vi "VF Laser Engine.vi"(0 "VF Laser Notifier":string="Not a Name", 11 "COM Port":string[](array[string])) -> ()   [LabVIEW 2020]
uses:
  Laser Controls/Laser Status.ctl
  Laser Controls/Laser Notifier Element.ctl
  Laser Controls/Laser Actions.ctl
  Laser Controls/Laser Settings.ctl
  Laser Controls/Laser Parameters.ctl
  <vilib>/Instr/_visa.llb/VISA Configure Serial Port (Instr).vi
panel:
  out "Startup Error":errorcluster
  in  "Get Power":bool
  out "Status":T1
  out "Light Emission?":bool
  out "Enabled (Interlock)?":bool
  in  "Get Status":bool
  in  "Laser Power (mW)":dbl
  in  "Laser On/Off":bool
  in  "Quit":bool
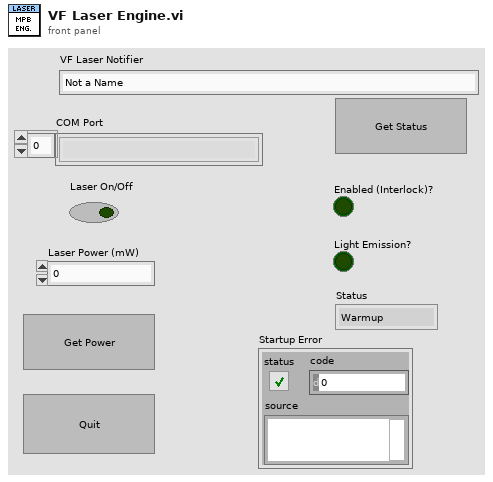
[diagram p1: front panel]
types:
  T1 = typedef "Laser Status.ctl" = enum16{"Warmup", "Ready", "Emission", "Tuning", "Error"}
  T2 = typedef "Laser Notifier Element.ctl" = cluster{"Laser Action":T3, "Received?":bool, "Enabled (Interlock)?":bool, "Light Emission?":bool, "Power (mW)":dbl, "Settings":T4, "Status":T1, "Error":errorcluster}
  T3 = typedef "Laser Actions.ctl" = enum16{"Error Check", "Set On/Off", "Set Power", "Set Parameter", "Get Power", "Get Status", "Get Parameter", "Quit"}
  T4 = typedef "Laser Settings.ctl" = cluster{"Laser Parameters":T5, "Value":dbl}
  T5 = typedef "Laser Parameters.ctl" = enum16{"Wavelength (nm)", "Pulsing?", "Rep. Rate", "External Control"}
  T6 = enum32{"Invalid", "Standard", "Closed", "Hidden", "Minimized", "Maximized"}
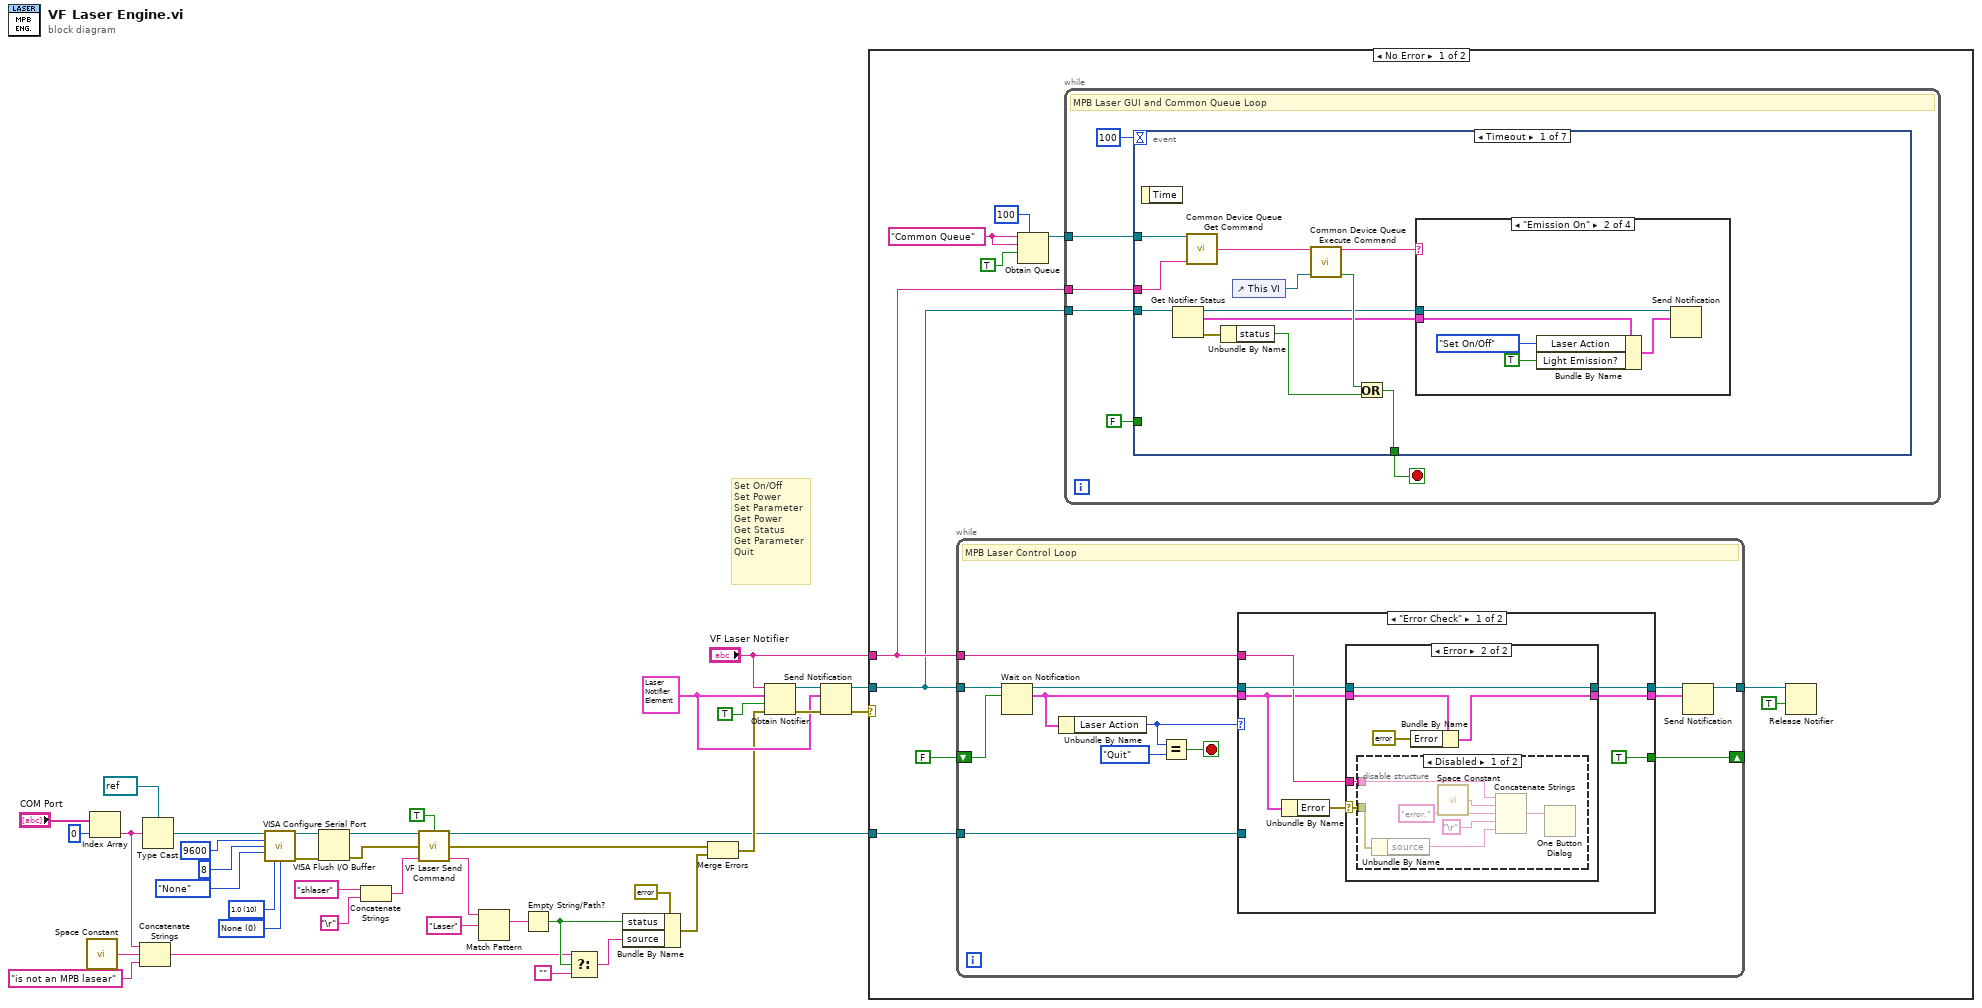
[diagram p0: block diagram]
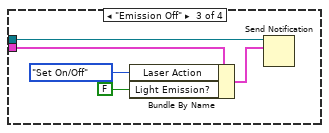
[diagram p3: hidden frame]
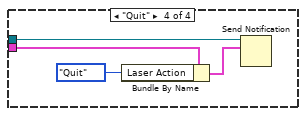
[diagram p4: hidden frame]
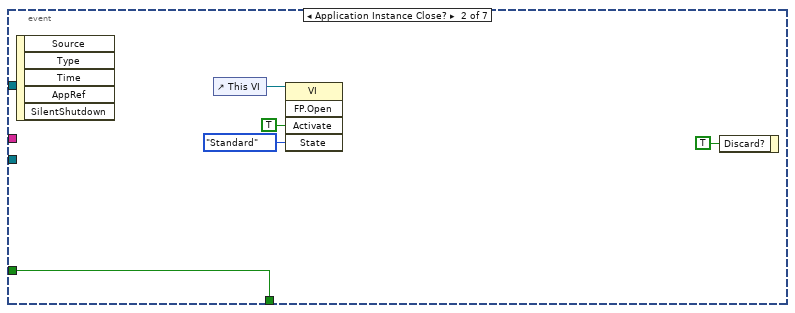
[diagram p5: hidden frame]
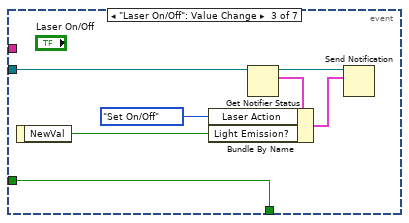
[diagram p6: hidden frame]
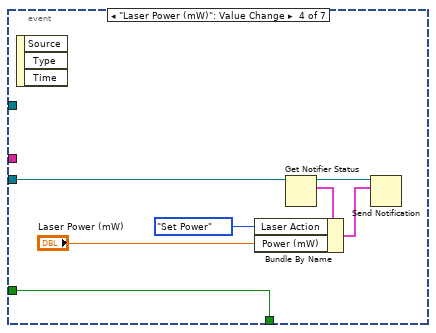
[diagram p7: hidden frame]
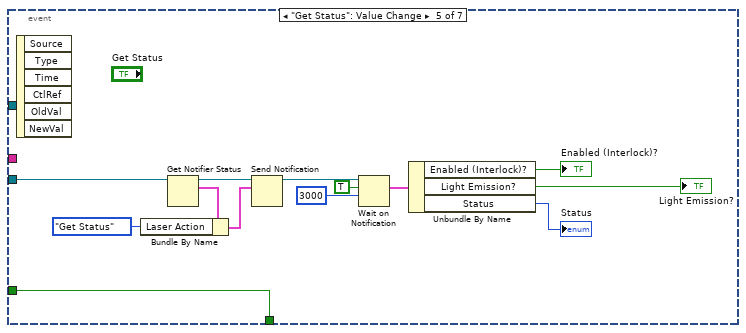
[diagram p8: hidden frame]
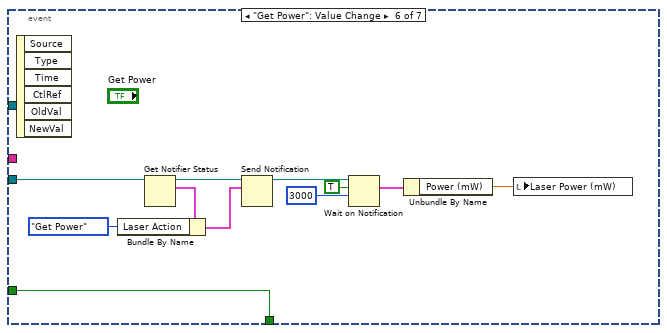
[diagram p9: hidden frame]
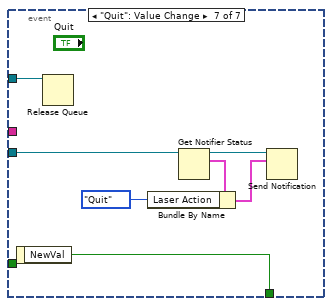
[diagram p10: hidden frame]
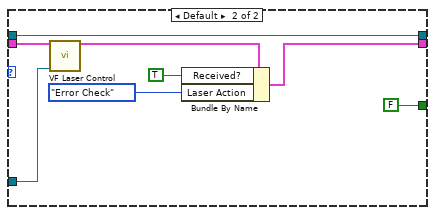
[diagram p13: hidden frame]
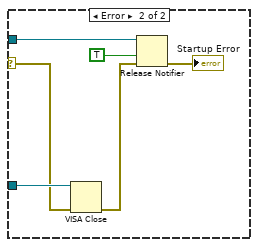
[diagram p14: hidden frame]
diagram:
  w25 = T2 {"Laser Action"=enum."Get Status", "Received?"=FALSE, "Enabled (Interlock)?"=FALSE, "Light Emission?"=FALSE, "Power (mW)"=0.0, "Settings"={"Laser Parameters"=enum."Wavelength (nm)", "Value"=0.0}, "Status"=enum."Error", "Error"={"status"=FALSE, "code"=0, "source"=""}} ("Laser Notifier Element")
  w30 = u16 0 items=["None", "XON/XOFF", "RTS/CTS", "XON/XOFF & RTS/CTS", "DTR/DSR", "XON/XOFF & DTR/DSR"] ("flow control (0:none)")
  w29 = u16 10 items=["1.0"=10, "1.5"=15, "2.0"=20] ("stop bits (10: 1 bit)")
  # "Set On/Off\nSet Power\nSet Parameter\nGet Power\nGet Status\nGet Parameter\nQuit"
  n1 = call <vilib>:"Space Constant.vi"() -> ("String"=w7:string)
  n2 = Index Array(array="COM Port", index=0) -> (element=w8:string)
  n3 = Concatenate Strings(w8, w7, "is not an MPB lasear" ("string")) -> (w4:string)
  n4 = Type Cast(type=refnum<visa-resource-name> refnum ("VISA resource name"), x=w8) -> (*(type *) &x=w22:refnum<visa-resource-name>)
  n5 = call-poly "VISA Configure Serial Port"("VISA resource name"=w22, "baud rate (9600)"=u32 9600, "data bits (8)"=u16 8, "parity (0:none)"=enum16{"None", "Odd", "Even", "Mark", "Space"}."None", "stop bits (10: 1 bit)"=w29, "flow control (0:none)"=w30) -> ("VISA resource name out"=w24:refnum<visa-resource-name>, "error out"=w23:errorcluster)  [unwired: 8 in]
  n6 = VISA Flush I/O Buffer(VISA resource name=w24, error in (no error)=w23) -> (VISA resource name out=w21:refnum<visa-resource-name>, error out=w19:errorcluster)  [unwired: 1 in]
  n7 = Concatenate Strings("shlaser", "\r") -> (w16:string)
  n8 = call "VF Laser Send Command.vi"("VISA Ref"=w21, "Wait for Reply?"=TRUE, "Error In"=w19, "Command"=w16) -> ("VISA Ref Out"=w11:refnum<visa-resource-name>, "Error Out"=w13:errorcluster, "Response"=w15:string)  [unwired: 9 in]
  n9 = Match Pattern(string=w15, regular expression="Laser") -> (match substring=w10:string)  [unwired: 1 in, 3 out]
  n10 = Empty String/Path?(string/path=w10) -> (empty?=w5:bool)
  n11 = Select(t=w4, s=w5, f="") -> (s? t:f=w3:string)
  n12 = Bundle By Name(cluster=errorcluster {"status"=FALSE, "code"=0, "source"=""} ("error in"), "status"=w5, "source"=w3) -> (w1:errorcluster)
  n13 = Merge Errors(w13, w1) -> (w12:errorcluster)
  n14 = Obtain Notifier(name (unnamed)="VF Laser Notifier", notification data type=w25, create if not found? (T)=TRUE, error in (no error)=w12) -> (notifier out=w38:refnum<notifier>, error out=w37:errorcluster)  [unwired: 1 out]
  n15 = Send Notification(notification=w25, notifier=w38, error in (no error)=w37) -> (notifier out=w36:refnum<notifier>, error out=w35:errorcluster)
  n16 = case shown="No Error" w35 {
    selector: w35 -> [_ w176]
    tunnel: w36 -> [w41 w178]
    tunnel: "VF Laser Notifier" -> [w42 _]
    tunnel: w11 -> [w40 w177]
    frame No Error {
      w46 = "Common Queue" ("Unique Notifier Name")
      n17 = while {
        tunnel: w41 -> [w142]
        tunnel: [w143] -> w48
        shift-right: [w135] -> _
        shift-left: FALSE -> [w137]
        tunnel: w42 -> [w134]
        tunnel: w40 -> [w132]
        stop <- w144 stop-if-true
        # "MPB Laser Control Loop"
        n18 = Wait on Notification(notifier=w142, ignore previous (F)=w137) -> (notifier out=w141:refnum<notifier>, notification=w140:T2)  [unwired: 2 in, 2 out]
        n19 = Unbundle By Name(w140) -> ("Laser Action"=w139:T3)
        n20 = Equal?(x=w139, y=Laser_Actions."Quit") -> (x = y?=w144:bool)
        n21 = case shown="\"Error Check\"" w139 {
          tunnel: w141 -> [w151 w167]
          tunnel: [w150 w167] -> w138
          tunnel: w140 -> [w147 w169]
          tunnel: w134 -> [w149 _]
          tunnel: [w148 w173] -> w136
          tunnel: [TRUE FALSE] -> w135
          tunnel: w132 -> [_ w174]
          frame "Error Check" {
            n22 = Unbundle By Name(w147) -> ("Error"=w146:errorcluster)
            n23 = case shown="Error" w146 {
              selector: w146 -> [_ w155]
              tunnel: w147 -> [w152 w159]
              tunnel: [w153 w157] -> w150
              tunnel: w151 -> [w153 w157]
              tunnel: w149 -> [_ w154]
              tunnel: [w152 w156] -> w148
              frame No Error {
              }
              frame Error {
                n24 = disable-structure shown="Disabled" {
                  disable-tunnel: w155 -> [w163 _]
                  disable-tunnel: w154 -> [w162 _]
                  frame Disabled {
                    n25 = Unbundle By Name(w163) -> ("source"=w161:string)
                    n26 = call <vilib>:"Space Constant.vi"() -> ("String"=w166:string)
                    n27 = Concatenate Strings(w162, w166, "error." ("string"), "\r", w161) -> (w164:string)
                    n28 = One Button Dialog(message=w164) -> ()  [unwired: 1 in, 1 out]
                  }
                  frame Enabled {
                  }
                }
                n29 = Bundle By Name(cluster=w159, "Error"=errorcluster {"status"=FALSE, "code"=0, "source"=""}) -> (w156:T2)
              }
            }
          }
          frame Default {
            n30 = call "VF Laser Control.vi"("Laser Notifier Element"=w169, "VISA Ref"=w174) -> ("Laser Notifier Element"=w168:T2)  [unwired: 13 in]
            n31 = Bundle By Name(cluster=w168, "Received?"=TRUE, "Laser Action"=Laser_Actions."Error Check") -> (w173:T2)
          }
        }
        n32 = Send Notification(notification=w136, notifier=w138) -> (notifier out=w143:refnum<notifier>)  [unwired: 1 in, 1 out]
      }
      n33 = Obtain Queue(max queue size (-1, unlimited)=100, name (unnamed)=w46, element data type=w46, create if not found? (T)=TRUE) -> (queue out=w43:refnum<queue>)  [unwired: 1 in, 2 out]
      n34 = while {
        tunnel: w43 -> [w54]
        tunnel: w42 -> [w52]
        tunnel: w41 -> [w53]
        stop <- w51 stop-if-true
        # "MPB Laser GUI and Common Queue Loop"
        n35 = event shown="[0] Timeout" {
          selector: _ -> [_ _ _ _ _ _ _]
          dyn-events: _ -> [_ _ _ _ _ _ _]
          timeout: 100 -> [_ _ _ _ _ _ _]
          tunnel: w54 -> [w61 _ _ _ _ _ w131]
          tunnel: w53 -> [w60 _ w88 w95 w109 w120 w130]
          tunnel: w52 -> [w59 _ _ _ _ _ _]
          tunnel: [w58 w86 w93 w100 w113 w124 w128] -> w51
          tunnel: FALSE -> [_ w86 w93 w100 w113 w124 _]
          event Timeout {
            n36 = event-data() -> ()  [unwired: 1 in, 1 out]
            n37 = Get Notifier Status(notifier=w60) -> (notifier out=w62:refnum<notifier>, current notification=w57:T2, error out=w67:errorcluster)  [unwired: 1 in, 2 out]
            n38 = call "Common Device Queue Get Command.vi"("Common Queue"=w61, "Notifier Name"=w59) -> ("Command"=w66:string)  [unwired: 12 in, 1 out]
            n39 = Unbundle By Name(w67) -> ("status"=w64:bool)
            n40 = control-ref of="This VI"() -> (w65:refnum<vi>)
            n41 = call "Common Device Queue Execute Command.vi"("Common Command"=w66, "VI Refnum"=w65) -> ("Common Command"=w56:string, "Quit?"=w63:bool)  [unwired: 12 in]
            n42 = Or(x=w63, y=w64) -> (x .or. y?=w58:bool)
            n43 = case shown="\"Emission On\"" w56 {
              tunnel: w62 -> [_ w72 w77 w81]
              tunnel: w57 -> [_ w71 w76 w80]
              frame Default {
              }
              frame "Emission On" {
                n44 = Bundle By Name(cluster=w71, "Laser Action"=Laser_Actions."Set On/Off", "Light Emission?"=TRUE) -> (w70:T2)
                n45 = Send Notification(notification=w70, notifier=w72) -> ()  [unwired: 1 in, 2 out]
              }
              frame "Emission Off" {
                n46 = Bundle By Name(cluster=w76, "Laser Action"=Laser_Actions."Set On/Off", "Light Emission?"=FALSE) -> (w75:T2)
                n47 = Send Notification(notification=w75, notifier=w77) -> ()  [unwired: 1 in, 2 out]
              }
              frame "Quit" {
                n48 = Bundle By Name(cluster=w80, "Laser Action"=Laser_Actions."Quit") -> (w79:T2)
                n49 = Send Notification(notification=w79, notifier=w81) -> ()  [unwired: 1 in, 2 out]
              }
            }
          }
          event Application Instance Close? {
            n50 = event-data() -> ()  [unwired: 1 in, 5 out]
            n51 = control-ref of="This VI"() -> (w83:refnum<vi>)
            n52 = invoke class="VI" method="FP.Open"(reference=w83, "Activate"=TRUE ("Activate?"), "State"=T6."Standard") -> ()  [unwired: 2 in, 5 out]
            n53 = event-data("Discard?"=TRUE) -> ()  [unwired: 1 in, 1 out]
          }
          event "Laser On/Off": Value Change {
            n54 = event-data() -> ("NewVal"=w87:bool)  [unwired: 1 in]
            n55 = Get Notifier Status(notifier=w88) -> (notifier out=w92:refnum<notifier>, current notification=w91:T2)  [unwired: 1 in, 3 out]
            n56 = Bundle By Name(cluster=w91, "Laser Action"=Laser_Actions."Set On/Off", "Light Emission?"=w87) -> (w89:T2)
            n57 = Send Notification(notification=w89, notifier=w92) -> ()  [unwired: 1 in, 2 out]
          }
          event "Laser Power (mW)": Value Change {
            n58 = event-data() -> ()  [unwired: 1 in, 3 out]
            n59 = Get Notifier Status(notifier=w95) -> (notifier out=w99:refnum<notifier>, current notification=w98:T2)  [unwired: 1 in, 3 out]
            n60 = Bundle By Name(cluster=w98, "Laser Action"=Laser_Actions."Set Power", "Power (mW)"="Laser Power (mW)") -> (w96:T2)
            n61 = Send Notification(notification=w96, notifier=w99) -> ()  [unwired: 1 in, 2 out]
          }
          event "Get Status": Value Change {
            n62 = event-data() -> ()  [unwired: 1 in, 6 out]
            n63 = Get Notifier Status(notifier=w109) -> (notifier out=w112:refnum<notifier>, current notification=w111:T2)  [unwired: 1 in, 3 out]
            n64 = Bundle By Name(cluster=w111, "Laser Action"=Laser_Actions."Get Status") -> (w110:T2)
            n65 = Send Notification(notification=w110, notifier=w112) -> (notifier out=w108:refnum<notifier>)  [unwired: 1 in, 1 out]
            n66 = Wait on Notification(notifier=w108, ignore previous (F)=TRUE, timeout in ms (-1)=3000) -> (notification=w105:T2)  [unwired: 1 in, 3 out]
            n67 = Unbundle By Name(w105) -> ("Enabled (Interlock)?"=→"Enabled (Interlock)?":bool, "Light Emission?"=→"Light Emission?":bool, "Status"=→"Status":T1)
          }
          event "Get Power": Value Change {
            n68 = event-data() -> ()  [unwired: 1 in, 6 out]
            n69 = Get Notifier Status(notifier=w120) -> (notifier out=w123:refnum<notifier>, current notification=w122:T2)  [unwired: 1 in, 3 out]
            n70 = Bundle By Name(cluster=w122, "Laser Action"=Laser_Actions."Get Power") -> (w121:T2)
            n71 = Send Notification(notification=w121, notifier=w123) -> (notifier out=w119:refnum<notifier>)  [unwired: 1 in, 1 out]
            n72 = Wait on Notification(notifier=w119, ignore previous (F)=TRUE, timeout in ms (-1)=3000) -> (notification=w116:T2)  [unwired: 1 in, 3 out]
            n73 = Unbundle By Name(w116) -> ("Power (mW)"=w115:dbl)
            n74 = local write "Laser Power (mW)"(w115) -> ()
          }
          event "Quit": Value Change {
            n75 = event-data() -> ("NewVal"=w128:bool)  [unwired: 1 in]
            n76 = Release Queue(queue=w131) -> ()  [unwired: 2 in, 3 out]
            n77 = Get Notifier Status(notifier=w130) -> (notifier out=w129:refnum<notifier>, current notification=w127:T2)  [unwired: 1 in, 3 out]
            n78 = Bundle By Name(cluster=w127, "Laser Action"=Laser_Actions."Quit") -> (w125:T2)
            n79 = Send Notification(notification=w125, notifier=w129) -> ()  [unwired: 1 in, 2 out]
          }
        }
      }
      n80 = Release Notifier(notifier=w48, force destroy? (F)=TRUE) -> ()  [unwired: 1 in, 3 out]
    }
    frame Error {
      n81 = VISA Close(VISA resource name=w177, error in (no error)=w176) -> (error out=w179:errorcluster)
      n82 = Release Notifier(notifier=w178, force destroy? (F)=TRUE, error in (no error)=w179) -> (error out=→"Startup Error":errorcluster)  [unwired: 2 out]
    }
  }
